vi "GPS VISA Test ON-OFF.vi"() -> ()   [LabVIEW 2009]
uses:
  <vilib>/Instr/_visa.llb/VISA Configure Serial Port (Instr).vi
panel:
  out "timeouts":dbl=1.0
  out "Success?":bool
  out "Output Halted":bool
  out "error out":errorcluster
  out "Timeout":bool
  out "concatenated string":string
  in  "stop button":bool
  in  "Stop":bool
  in  "Start":bool
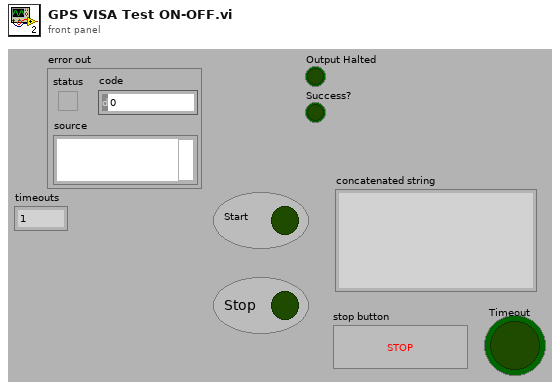
[diagram p1: front panel]
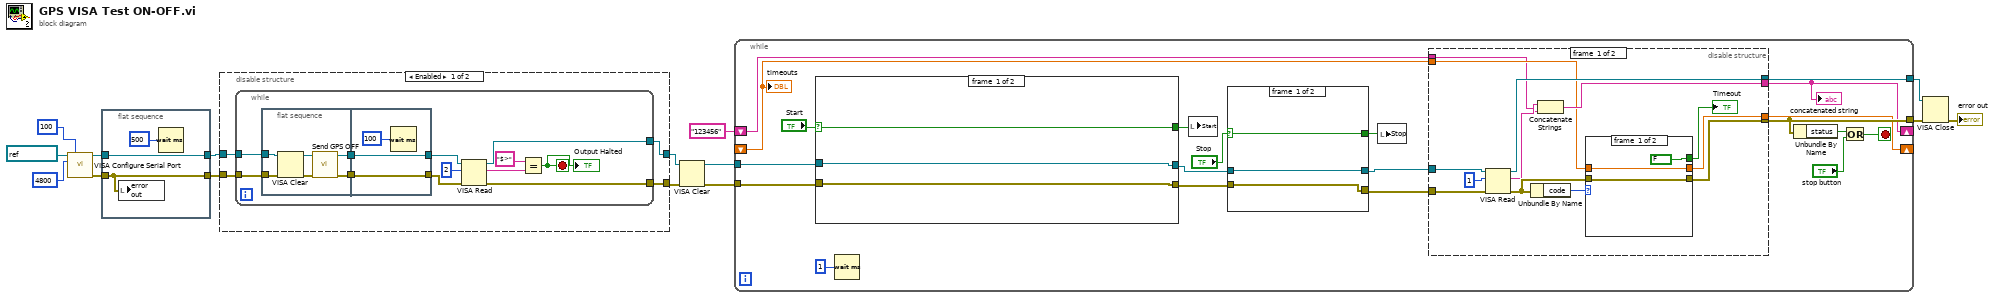
[diagram p0: block diagram]
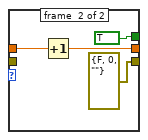
[diagram p3: hidden frame]
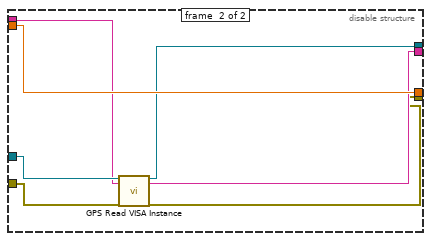
[diagram p4: hidden frame]
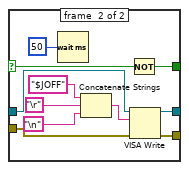
[diagram p5: hidden frame]
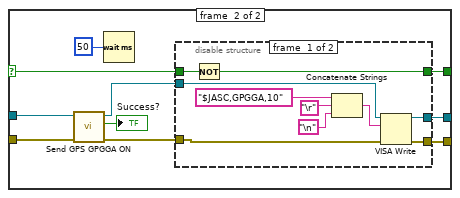
[diagram p6: hidden frame]
diagram:
  n1 = call-poly "VISA Configure Serial Port"("VISA resource name"=refnum<visa-resource-name> "COM1", "timeout (10sec)"=u32 100, "baud rate (9600)"=u32 4800) -> ("VISA resource name out"=w7:refnum<visa-resource-name>, "error out"=w12:errorcluster)  [unwired: 11 in]
  n2 = flat-sequence {
    tunnel: [w16] -> w6
    tunnel: w12 -> [w16]
    tunnel: w7 -> [w17]
    tunnel: [w17] -> w5
    frame #0 {
      n3 = local write "error out"(w16) -> ()
      n4 = Wait (ms)(milliseconds to wait=u32 500) -> ()  [unwired: 1 out]
    }
  }
  n5 = disable-structure shown="Enabled" {
    disable-tunnel: w6 -> [w22 w44]
    disable-tunnel: w5 -> [w21 w45]
    disable-tunnel: [w20 w44] -> w2
    disable-tunnel: [w19 w45] -> w1
    frame #0 {
      n6 = while {
        tunnel: w22 -> [w34]
        tunnel: w21 -> [w33]
        tunnel: [w28] -> w20
        tunnel: [w27] -> w19
        stop <- w29 stop-if-true
        n7 = flat-sequence {
          tunnel: w34 -> [w38]
          tunnel: w33 -> [w37]
          tunnel: [w36] -> w25
          tunnel: [w35] -> w23
          tunnel: [w42] -> w26
          tunnel: w25 -> [w42]
          tunnel: [w41] -> w24
          tunnel: w23 -> [w41]
          frame #0 {
            n8 = VISA Clear(VISA resource name=w37, error in (no error)=w38) -> (VISA resource name out=w40:refnum<visa-resource-name>, error out=w39:errorcluster)
            n9 = call "Send GPS OFF.vi"("error in (no error)"=w39, "VISA resource name"=w40) -> ("error out"=w36:errorcluster, "VISA resource name out"=w35:refnum<visa-resource-name>)  [unwired: 8 in]
          }
          frame #1 {
            n10 = Wait (ms)(milliseconds to wait=u32 100) -> ()  [unwired: 1 out]
          }
        }
        n11 = VISA Read(VISA resource name=w24, byte count=u32 2, error in (no error)=w26) -> (VISA resource name out=w27:refnum<visa-resource-name>, read buffer=w31:string, error out=w28:errorcluster)  [unwired: 1 out]
        n12 = Equal?(x="$>" ("read buffer"), y=w31) -> (x = y?=w29:bool)
        "Output Halted" <- w29
      }
    }
    frame #1 {
    }
  }
  n13 = VISA Clear(VISA resource name=w1, error in (no error)=w2) -> (VISA resource name out=w4:refnum<visa-resource-name>, error out=w3:errorcluster)
  n14 = while {
    tunnel: [w55] -> w13
    shift-right: [w46] -> _
    shift-left: "123456" ("Ascii to write 2") -> [w54]
    tunnel: [w51] -> w9
    tunnel: w4 -> [w50]
    tunnel: w3 -> [w49]
    shift-right: [w48] -> _
    shift-left: _ -> [w47]
    stop <- w58 stop-if-true
    n15 = case shown="True" "Start" {
      selector: "Start" -> [w109 w110]
      tunnel: [w107 w119] -> w63
      tunnel: [w108 w118] -> w60
      tunnel: [w109 w117] -> w62
      tunnel: w50 -> [w107 w115]
      tunnel: w49 -> [w108 w114]
      frame #0 {
      }
      frame #1 {
        n16 = call "Send GPS GPGGA ON.vi"("error in (no error)"=w114, "VISA resource name"=w115) -> ("error out"=w112:errorcluster, "Success?"=→"Success?":bool, "VISA resource name out"=w113:refnum<visa-resource-name>)  [unwired: 7 in]
        n17 = Wait (ms)(milliseconds to wait=u32 50) -> ()  [unwired: 1 out]
        n18 = disable-structure shown="Enabled" {
          disable-tunnel: [w129 w131] -> w119
          disable-tunnel: [w128 w130] -> w118
          disable-tunnel: [w127 _] -> w117
          disable-tunnel: w113 -> [w123 w131]
          disable-tunnel: w112 -> [w122 w130]
          disable-tunnel: w110 -> [w121 _]
          frame #0 {
            n19 = Not(x=w121) -> (.not. x?=w127:bool)
            n20 = Concatenate Strings("$JASC,GPGGA,10" ("Ascii to write 2"), "\r", "\n") -> (w124:string)
            n21 = VISA Write(VISA resource name=w123, write buffer=w124, error in (no error)=w122) -> (VISA resource name out=w129:refnum<visa-resource-name>, error out=w128:errorcluster)  [unwired: 1 out]
          }
          frame #1 {
          }
        }
      }
    }
    n22 = Wait (ms)(milliseconds to wait=u32 1) -> ()  [unwired: 1 out]
    n23 = local write "Start"(w62) -> ()
    n24 = case shown="False" "Stop" {
      selector: "Stop" -> [w94 w102]
      tunnel: w63 -> [w95 w106]
      tunnel: [w95 w105] -> w57
      tunnel: [w93 w104] -> w56
      tunnel: [w94 w103] -> w61
      tunnel: w60 -> [w93 w100]
      frame #0 {
      }
      frame #1 {
        n25 = Wait (ms)(milliseconds to wait=u32 50) -> ()  [unwired: 1 out]
        n26 = Concatenate Strings("$JOFF" ("Ascii to write 2"), "\r", "\n") -> (w98:string)
        n27 = Not(x=w102) -> (.not. x?=w103:bool)
        n28 = VISA Write(VISA resource name=w106, write buffer=w98, error in (no error)=w100) -> (VISA resource name out=w105:refnum<visa-resource-name>, error out=w104:errorcluster)  [unwired: 1 out]
      }
    }
    n29 = local write "Stop"(w61) -> ()
    n30 = disable-structure shown="Enabled" {
      disable-tunnel: w57 -> [w78 w90]
      disable-tunnel: w56 -> [w77 w92]
      disable-tunnel: [w75 w88] -> w55
      disable-tunnel: w54 -> [w66 w89]
      disable-tunnel: [w74 w87] -> w46
      disable-tunnel: [w70 w86] -> w51
      disable-tunnel: [w69 w91] -> w48
      disable-tunnel: w47 -> [w68 w91]
      frame #0 {
        n31 = VISA Read(VISA resource name=w78, byte count=u32 1, error in (no error)=w77) -> (VISA resource name out=w75:refnum<visa-resource-name>, read buffer=w67:string, error out=w72:errorcluster)  [unwired: 1 out]
        n32 = Unbundle By Name(w72) -> ("code"=w73:i32)
        n33 = Concatenate Strings(w67, w66) -> (w74:string)
        n34 = case shown="-1073807339" w73 {
          tunnel: w72 -> [w81 _]
          tunnel: [w81 errorcluster {"status"=FALSE, "code"=0, "source"=""} ("error out")] -> w70
          tunnel: [FALSE ("status") TRUE ("status")] -> w71
          tunnel: [w79 w83] -> w69
          tunnel: w68 -> [w79 w82]
          frame #0 {
          }
          frame #1 {
            n35 = Increment(x=w82) -> (x+1=w83:dbl)
          }
        }
        "Timeout" <- w71
      }
      frame #1 {
        n36 = call "GPS Read VISA Instance.vi"("VISA In"=w90, "Buffer In"=w89, "Error In"=w92) -> ("VISA Out"=w88:refnum<visa-resource-name>, "Buffer Out"=w87:string, "Error Out"=w86:errorcluster)  [unwired: 10 in, 4 out]
      }
    }
    "concatenated string" <- w46
    n37 = Unbundle By Name(w51) -> ("status"=w52:bool)
    n38 = Or(x=w52, y="stop button") -> (x .or. y?=w58:bool)
    "timeouts" <- w47
  }
  n39 = VISA Close(VISA resource name=w13, error in (no error)=w9) -> (error out=→"error out":errorcluster)
